vi "Claster.vi"() -> ()   [LabVIEW 2020]
panel:
  out "error out":errorcluster
  in  "error in":errorcluster
  in  "Wathe  Dtar":T1
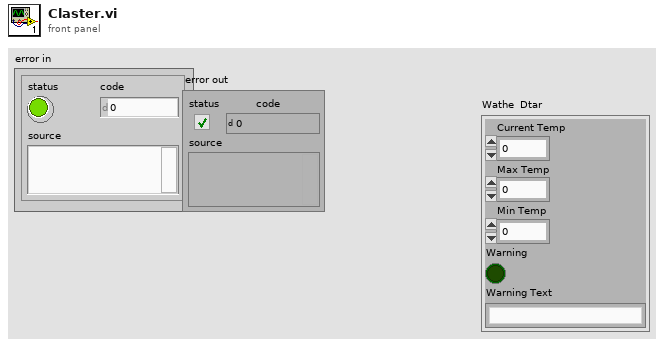
[diagram p1: front panel]
types:
  T1 = cluster{"Current Temp":dbl, "Max Temp":dbl, "Min Temp":dbl, "Warning":bool, "Warning Text":string}
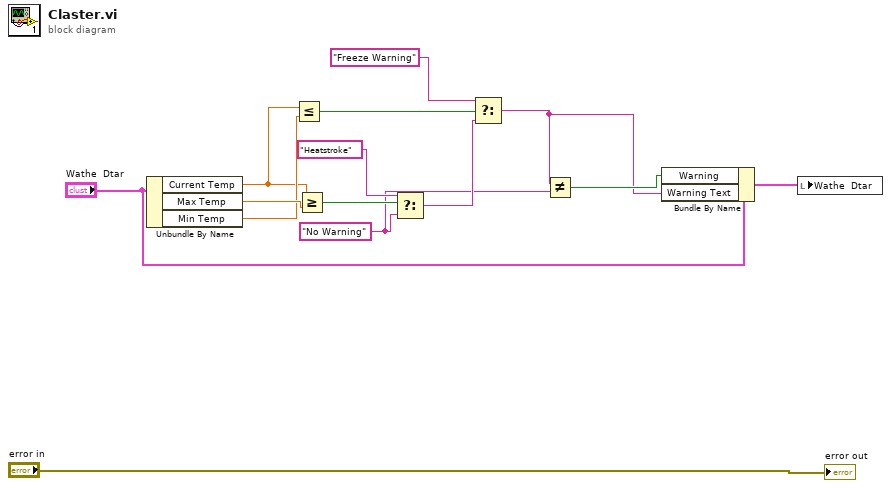
[diagram p0: block diagram]
diagram:
  w5 = "No Warning"
  n1 = Unbundle By Name("Wathe  Dtar") -> ("Current Temp"=w7:dbl, "Max Temp"=w13:dbl, "Min Temp"=w8:dbl)
  n2 = Less Or Equal?(x=w7, y=w8) -> (x <= y?=w6:bool)
  n3 = Greater Or Equal?(x=w7, y=w13) -> (x >= y?=w12:bool)
  n4 = Select(t="Heatstroke", s=w12, f=w5) -> (s? t:f=w10:string)
  n5 = Select(t="Freeze Warning", s=w6, f=w10) -> (s? t:f=w2:string)
  n6 = Not Equal?(x=w2, y=w5) -> (x != y?=w3:bool)
  n7 = Bundle By Name(cluster="Wathe  Dtar", "Warning"=w3, "Warning Text"=w2) -> (w1:T1)
  n8 = local write "Wathe  Dtar"(w1) -> ()
  "error out" <- "error in"
